vi "SysDef Launcher.vi"() -> ()   [LabVIEW 2014]
uses:
  NationalInstruments.VeriStand.Internal
  <vilib>/NI VeriStand/Execution/Workspace/NI_VS Workspace ExecutionAPI.lvlib
  <vilib>/NI Veristand/Execution/Project/NI_VS Project ExecutionAPI.lvlib
  NationalInstruments.VeriStand
panel:
  out "State":string
  in  "Stop":bool
  in  "Start":bool
  in  "System Definition File":path
  in  "Active Display":string(combo)
  in  "NIVS.App.Command":refnum<user-event>
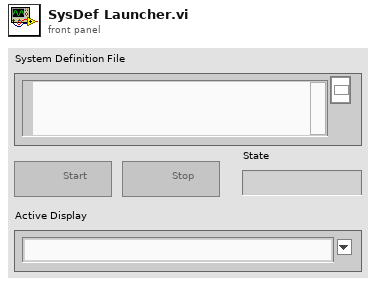
[diagram p1: front panel]
types:
  T1 = typedef "NI_VS Workspace ExecutionAPI.lvlib/WorkspaceAPI.ctl" = refnum<k24>
  T2 = typedef "NI_VS Workspace ExecutionAPI.lvlib/SystemStateEventRef.ctl" = cluster{"CustDatRef":refnum<user-event>, "EvtRef":refnum<k27>}
  T3 = typedef "NI_VS Workspace ExecutionAPI.lvlib/SystemStateRegEventRef.ctl" = refnum<event-registration>
  T4 = cluster{"Event Registration Refnum":refnum<event-registration>, "SystemChangeEventRef":T3}
  T5 = enum8{"Enabled", "Disabled", "Disabled and Grayed Out"}
  T6 = typedef "NI_VS Project ExecutionAPI.lvlib/Project Ref.ctl" = refnum<k24>
  T7 = typedef "NI_VS Workspace ExecutionAPI.lvlib/SystemState.ctl" = u8
  T8 = enum32{"invalid app kind", "Development System", "Run Time System", "Student Edition", "Embedded LabVIEW", "Evaluation", "Custom"}
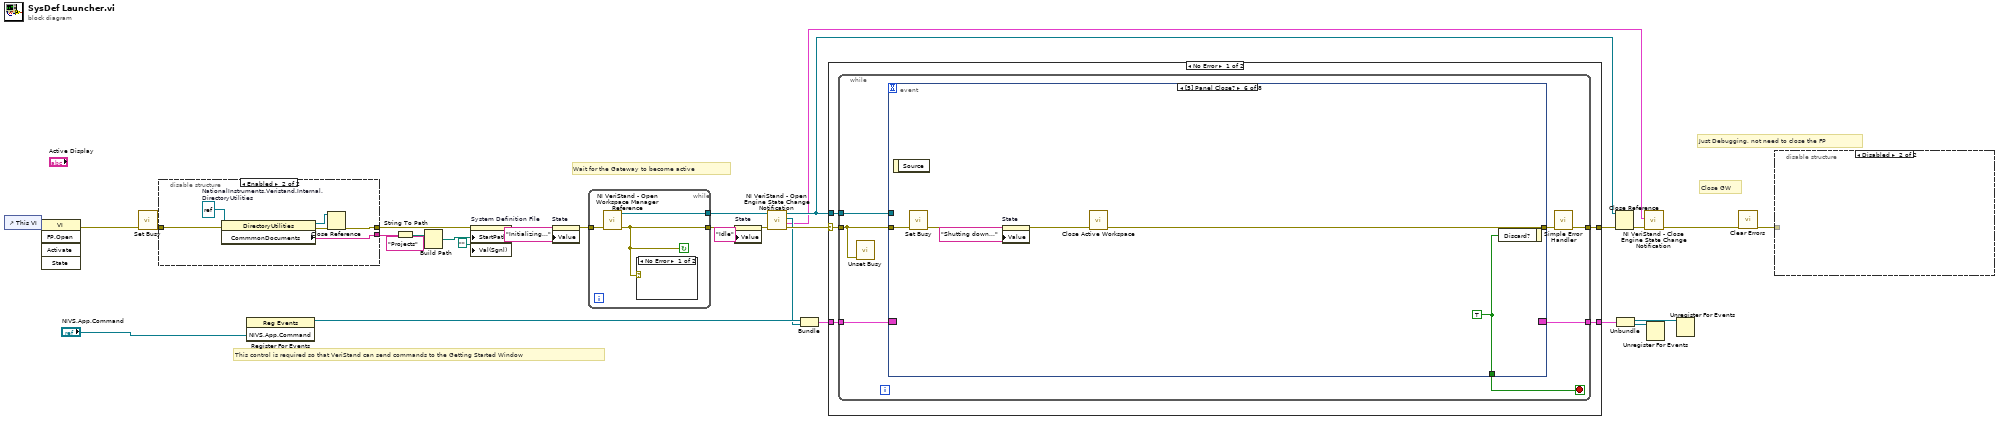
[diagram p0: block diagram]
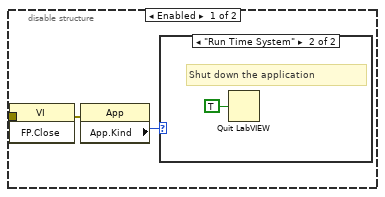
[diagram p2: hidden frame]
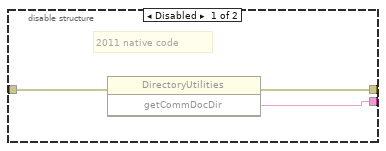
[diagram p4: hidden frame]
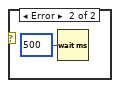
[diagram p5: hidden frame]
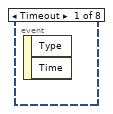
[diagram p6: hidden frame]
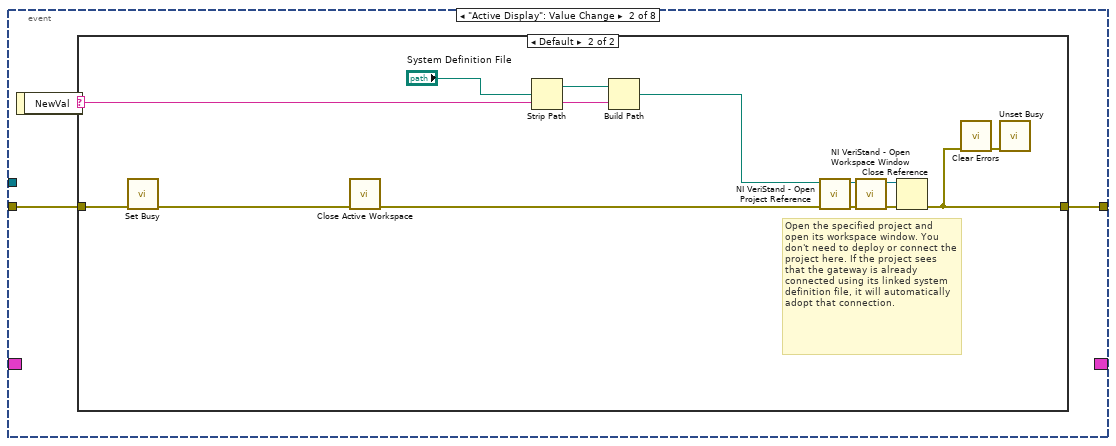
[diagram p7: hidden frame]
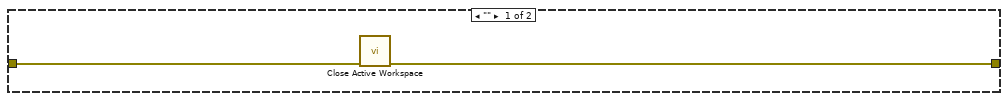
[diagram p8: hidden frame]
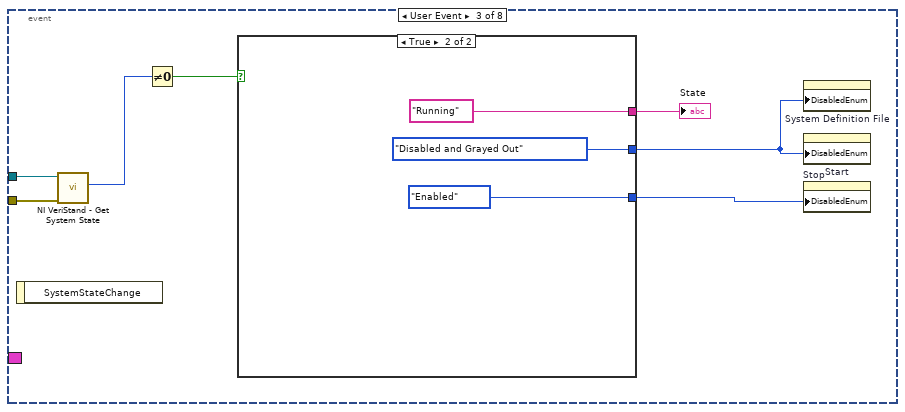
[diagram p9: hidden frame]
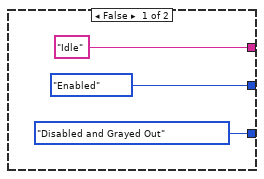
[diagram p10: hidden frame]
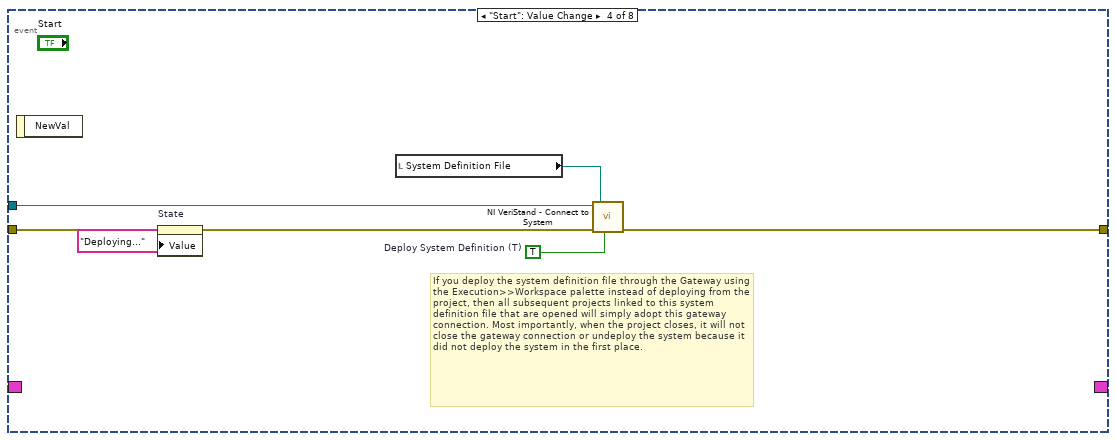
[diagram p11: hidden frame]
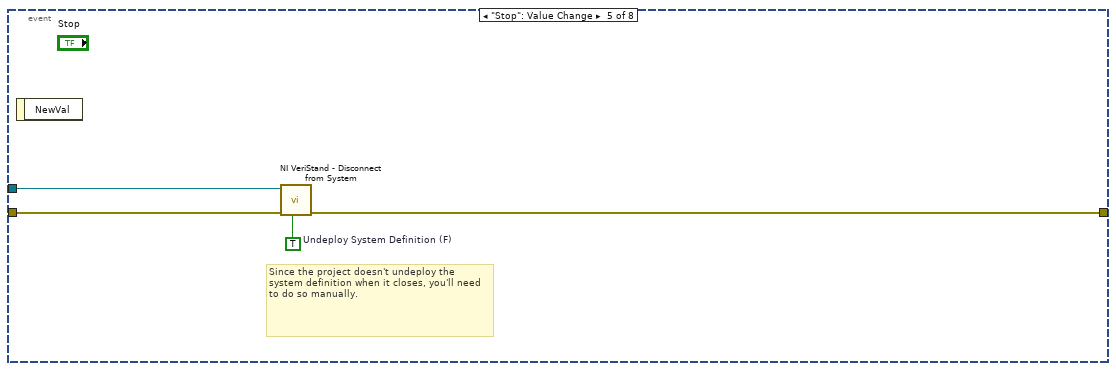
[diagram p12: hidden frame]
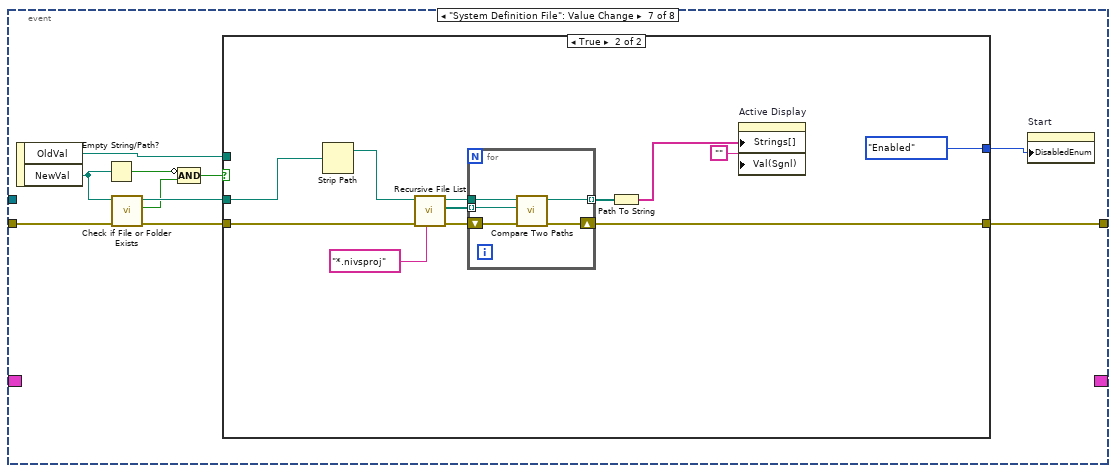
[diagram p13: hidden frame]
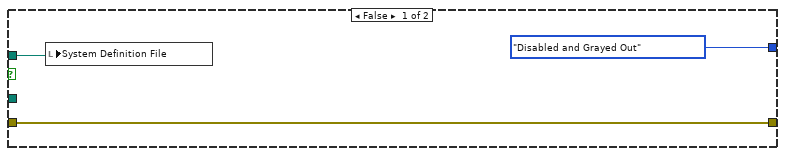
[diagram p14: hidden frame]
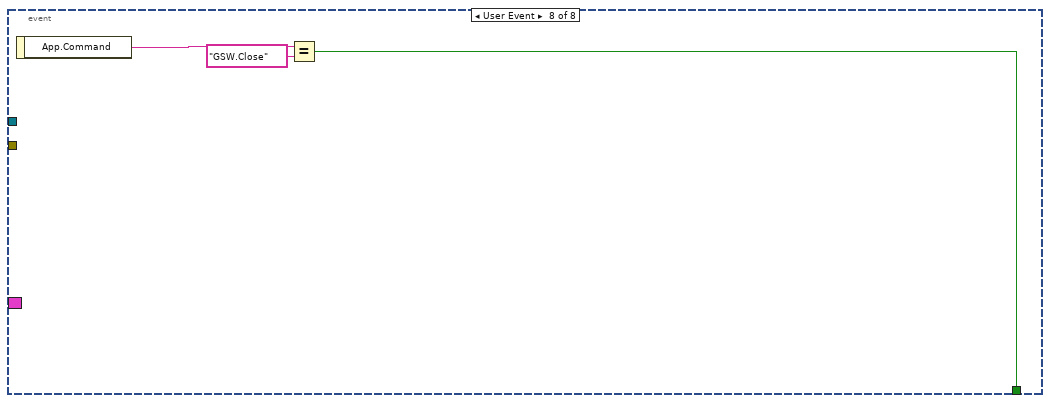
[diagram p15: hidden frame]
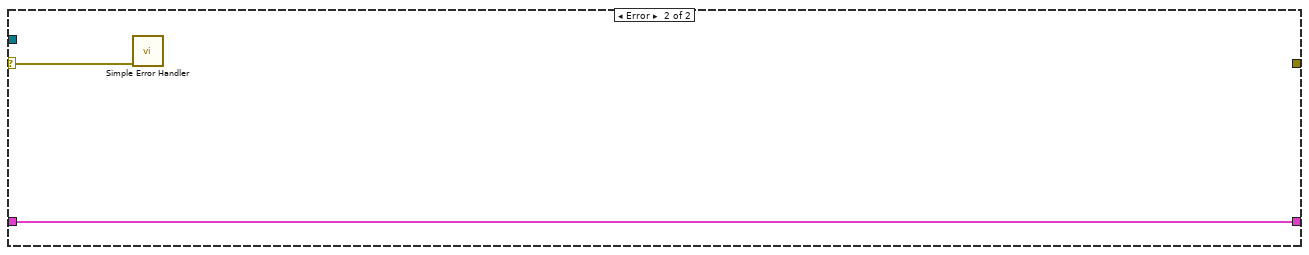
[diagram p16: hidden frame]
diagram:
  # "Close GW"
  # "Just Debugging, not need to close the FP"
  # "This control is required so that VeriStand can send commands to the Getting Started Window"
  # "Wait for the Gateway to become active"
  n1 = control-ref of="This VI"() -> (w29:refnum<vi>)
  n2 = invoke class="VI" method="FP.Open"(reference=w29) -> (error out=w2:errorcluster)  [unwired: 4 in, 4 out]
  n3 = call <vilib>:"Set Busy.vi"("error in (no error)"=w2) -> ("error out"=w4:errorcluster)  [unwired: 9 in, 1 out]
  n4 = disable-structure shown="Enabled" {
    disable-tunnel: [w33 w36] -> w27
    disable-tunnel: [w32 w38] -> w5
    disable-tunnel: w4 -> [w31 w35]
    frame Disabled {
      # "2011 native code"
      n5 = invoke class="DirectoryUtilities" method="getCommDocDir"(error in=w31) -> (error out=w32:errorcluster, "getCommDocDir"=w33:string)  [unwired: 2 in, 1 out]
    }
    frame Enabled {
      w34 = refnum<k24> refnum  # NationalInstruments.Veristand.Internal.DirectoryUtilities
      n6 = property class="DirectoryUtilities"(reference=w34, error in=w35) -> (reference out=w39:refnum<k24>, error out=w37:errorcluster, "CommmonDocuments"=w36:string)
      n7 = Close Reference(reference=w39, error in (no error)=w37) -> (error out=w38:errorcluster)
    }
  }
  n8 = register-events("NIVS.App.Command") -> (reference out=w21:refnum<event-registration>)  [unwired: 2 in, 1 out]
  n9 = String To Path(string=w27) -> (path=w26:path)
  n10 = Build Path(base path=w26, name or relative path="Projects") -> (appended path=w24:path)
  n11 = property on="System Definition File" class="Path"(error in=w5, "StartPath"=w24, "Val(Sgnl)"=path "") -> (error out=w11:errorcluster)  [unwired: 1 in, 1 out]
  n12 = property on="State" class="Str"(error in=w11, "Value"="Initializing..." ("State")) -> (error out=w10:errorcluster)  [unwired: 1 in, 1 out]
  n13 = while {
    tunnel: w10 -> [w42]
    tunnel: [w41] -> w22
    tunnel: [w40] -> w7
    stop <- w40 continue-if-true
    n14 = call <vilib>:"NI VeriStand - Open Workspace Manager Reference.vi"("error in (no error)"=w42) -> ("error out"=w40:errorcluster, "WorkspaceManager"=w41:T1)  [unwired: 9 in]
    n15 = case shown="No Error" w40 {
      frame No Error {
      }
      frame Error {
        n16 = Wait (ms)(milliseconds to wait=u32 500) -> ()  [unwired: 1 out]
      }
    }
  }
  n17 = property on="State" class="Str"(error in=w7, "Value"="Idle" ("State")) -> (error out=w6:errorcluster)  [unwired: 1 in, 1 out]
  n18 = call <vilib>:"NI VeriStand - Open Engine State Change Notification.vi"("error in (no error)"=w6, "WorkspaceManager in"=w22) -> ("error out"=w30:errorcluster, "SystemStateRefs"=w14:T2, "SystemChangeEventRef"=w19:T3, "WorkspaceManager out"=w18:T1)  [unwired: 6 in]
  n19 = Bundle("Event Registration Refnum"=w21, "SystemChangeEventRef"=w19) -> (w20:T4)  [unwired: 1 in]
  n20 = case shown="No Error" w30 {
    selector: w30 -> [w47 w137]
    tunnel: [w48 _] -> w23
    tunnel: w20 -> [w46 w138]
    tunnel: [w45 w138] -> w17
    tunnel: w18 -> [w44 _]
    frame No Error {
      n21 = while {
        tunnel: [w53] -> w48
        tunnel: w47 -> [w49]
        tunnel: w46 -> [w52]
        tunnel: [w51] -> w45
        tunnel: w44 -> [w50]
        stop <- w55 stop-if-true
        n22 = call <vilib>:"Unset Busy.vi"("error in (no error)"=w49) -> ()  [unwired: 10 in, 1 out]
        n23 = event shown="[5] Panel Close?" {
          selector: w52 -> [_ _ _ _ _ _ _ _]
          dyn-events: [_ _ _ _ _ _ _ _] -> w51
          timeout: _ -> [_ _ _ _ _ _ _ _]
          tunnel: [_ _ _ _ _ w103 _ w134] -> w55
          tunnel: [_ w58 _ w90 w94 w98 w105 _] -> w54
          tunnel: w49 -> [_ w57 w79 w88 w96 w100 w113 _]
          tunnel: w50 -> [_ _ w80 w91 w95 _ _ _]
          event Timeout {
            n24 = event-data() -> ()  [unwired: 1 in, 2 out]
          }
          event "Active Display": Value Change {
            n25 = event-data() -> ("NewVal"=w56:string)  [unwired: 1 in]
            n26 = case shown="Default" w56 {
              selector: w56 -> [_ w66]
              tunnel: [w59 w63] -> w58
              tunnel: w57 -> [w60 w65]
              frame "" {
                n27 = call "Close Active Workspace.vi"("error in (no error)"=w60) -> ("error out"=w59:errorcluster)  [unwired: 10 in]
              }
              frame Default {
                # "Open the specified project and open its workspace window. You don't need to deploy or connect the project here. If the project sees that the gateway is already connected using its linked system definition file, it will automatically adopt that connection."
                n28 = call <vilib>:"Set Busy.vi"("error in (no error)"=w65) -> ("error out"=w62:errorcluster)  [unwired: 9 in, 1 out]
                n29 = call "Close Active Workspace.vi"("error in (no error)"=w62) -> ("error out"=w61:errorcluster)  [unwired: 10 in]
                n30 = Strip Path(path="System Definition File") -> (stripped path=w70:path)  [unwired: 1 out]
                n31 = Build Path(base path=w70, name or relative path=w66) -> (appended path=w69:path)
                n32 = call <vilib>:"NI VeriStand - Open Project Reference.vi"("error in (no error)"=w61, "Project File Path"=w69) -> ("error out"=w68:errorcluster, "Project Ref"=w67:T6)  [unwired: 8 in]
                n33 = call <vilib>:"NI VeriStand - Open Workspace Window.vi"("error in (no error)"=w68, "Project Ref in"=w67) -> ("error out"=w73:errorcluster, "Project Ref out"=w72:T6)  [unwired: 8 in]
                n34 = Close Reference(reference=w72, error in (no error)=w73) -> (error out=w63:errorcluster)
                n35 = call <vilib>:"Clear Errors.vi"("error in (no error)"=w63) -> ("error out"=w64:errorcluster)  [unwired: 5 in, 1 out]
                n36 = call <vilib>:"Unset Busy.vi"("error in (no error)"=w64) -> ()  [unwired: 10 in, 1 out]
              }
            }
          }
          event User Event {
            n37 = event-data() -> ()  [unwired: 1 in, 1 out]
            n38 = call <vilib>:"NI VeriStand - Get System State.vi"("error in (no error)"=w79, "WorkspaceManager in"=w80) -> ("System State"=w78:T7)  [unwired: 5 in, 4 out]
            n39 = Not Equal To 0?(x=w78) -> (x != 0?=w77:bool)
            n40 = case shown="True" w77 {
              tunnel: ["Idle" ("State") "Running" ("State")] -> w74
              tunnel: [T5."Enabled" ("Disabled") T5."Disabled and Grayed Out" ("Disabled")] -> w75
              tunnel: [T5."Disabled and Grayed Out" ("Disabled") T5."Enabled" ("Disabled")] -> w76
              frame False {
              }
              frame True {
              }
            }
            "State" <- w74
            n41 = property on="System Definition File" class="Path"("DisabledEnum"=w75) -> ()  [unwired: 2 in, 2 out]
            n42 = property on="Start" class="Bool"("DisabledEnum"=w75) -> ()  [unwired: 2 in, 2 out]
            n43 = property on="Stop" class="Bool"("DisabledEnum"=w76) -> ()  [unwired: 2 in, 2 out]
          }
          event "Start": Value Change {
            w93 = TRUE  # Deploy System Definition (T)
            # "If you deploy the system definition file through the Gateway using the Execution>>Workspace palette instead of deploying from the project, then all subsequent projects linked to this system definition file that are opened will simply adopt this gateway connection. Most importantly, when the project closes, it will not close the gateway connection or undeploy the system because it did not deploy the system in the first place."
            n44 = event-data() -> ()  [unwired: 1 in, 1 out]
            n45 = property on="State" class="Str"(error in=w88, "Value"="Deploying..." ("State")) -> (error out=w87:errorcluster)  [unwired: 1 in, 1 out]
            n46 = local read "System Definition File"() -> (w92:path)
            n47 = call <vilib>:"NI VeriStand - Connect to System.vi"("Deploy System Definition (T)"=w93, "error in (no error)"=w87, "System Definition File (.nivssdf)"=w92, "WorkspaceManager in"=w91) -> ("error out"=w90:errorcluster)  [unwired: 6 in, 1 out]
          }
          event "Stop": Value Change {
            w97 = TRUE  # Undeploy System Definition (F)
            # "Since the project doesn't undeploy the system definition when it closes, you'll need to do so manually."
            n48 = event-data() -> ()  [unwired: 1 in, 1 out]
            n49 = call <vilib>:"NI VeriStand - Disconnect from System.vi"("Undeploy System Definition (F)"=w97, "error in (no error)"=w96, "WorkspaceManager in"=w95) -> ("error out"=w94:errorcluster)  [unwired: 7 in, 1 out]
          }
          event Panel Close? {
            w103 = TRUE
            n50 = event-data() -> ()  [unwired: 1 in, 1 out]
            n51 = call <vilib>:"Set Busy.vi"("error in (no error)"=w100) -> ("error out"=w99:errorcluster)  [unwired: 9 in, 1 out]
            n52 = property on="State" class="Str"(error in=w99, "Value"="Shutting down..." ("State")) -> (error out=w101:errorcluster)  [unwired: 1 in, 1 out]
            n53 = call "Close Active Workspace.vi"("error in (no error)"=w101) -> ("error out"=w98:errorcluster)  [unwired: 10 in]
            n54 = event-data("Discard?"=w103) -> ()  [unwired: 1 in, 1 out]
          }
          event "System Definition File": Value Change {
            n55 = event-data() -> ("OldVal"=w106:path, "NewVal"=w110:path)  [unwired: 1 in]
            n56 = Empty String/Path?(string/path=w110) -> (empty?=w108:bool)
            n57 = call <vilib>:"Check if File or Folder Exists.vi"("error in (no error)"=w113, "path"=w110) -> ("error out"=w112:errorcluster, "file or folder exists?"=w109:bool, "dup path"=w111:path)  [unwired: 7 in]
            n58 = Compound Arithmetic op=AND(invert w108, w109) -> (w107:bool)
            n59 = case shown="True" w107 {
              tunnel: w112 -> [w115 w128]
              tunnel: w111 -> [_ w127]
              tunnel: w106 -> [w116 _]
              tunnel: [w115 w118] -> w105
              tunnel: [T5."Disabled and Grayed Out" ("Disabled") T5."Enabled" ("Disabled")] -> w104
              frame False {
                n60 = local write "System Definition File"(w116) -> ()
              }
              frame True {
                n61 = Strip Path(path=w127) -> (stripped path=w126:path)  [unwired: 1 out]
                n62 = call <vilib>:"Recursive File List.vi"("pattern"="*.nivsproj", "error in (no error)"=w128, "Folder Path"=w126) -> ("error out"=w124:errorcluster, "All Files in Dir"=w123:path[], "dup Folder Path"=w122:path)  [unwired: 4 in, 2 out]
                n63 = for {
                  tunnel: w123 -> [w132] mode=indexing
                  tunnel: w122 -> [w131]
                  tunnel: [w130] -> w121 mode=indexing
                  shift-right: [w129] -> w118
                  shift-left: w124 -> [w133]
                  n64 = call <vilib>:"Compare Two Paths.vi"("error in (no error)"=w133, "Path 2"=w132, "Path 1"=w131) -> ("error out"=w129:errorcluster, "Relative Path from 1 to 2"=w130:path)  [unwired: 5 in, 2 out]
                }
                n65 = Path To String(path=w121) -> (string=w120:string[])
                n66 = property on="Active Display" class="CmbBox"("Strings[]"=w120, "Val(Sgnl)"="") -> ()  [unwired: 2 in, 2 out]
              }
            }
            n67 = property on="Start" class="Bool"("DisabledEnum"=w104) -> ()  [unwired: 2 in, 2 out]
          }
          event User Event {
            n68 = event-data() -> ("App.Command"=w136:string)  [unwired: 1 in]
            n69 = Equal?(x=w136, y="GSW.Close") -> (x = y?=w134:bool)
          }
        }
        n70 = call <vilib>:"Simple Error Handler.vi"("error in (no error)"=w54) -> ("error out"=w53:errorcluster)  [unwired: 4 in, 4 out]
      }
    }
    frame Error {
      n71 = call <vilib>:"Simple Error Handler.vi"("error in (no error)"=w137) -> ()  [unwired: 4 in, 5 out]
    }
  }
  n72 = Close Reference(reference=w18, error in (no error)=w23) -> (error out=w12:errorcluster)
  n73 = Unbundle(w17) -> ("Event Registration Refnum"=w15:refnum<event-registration>, "SystemChangeEventRef"=w16:T3)
  n74 = call <vilib>:"NI VeriStand - Close Engine State Change Notification.vi"("error in (no error)"=w12, "SystemStateRefs"=w14) -> ("error out"=w1:errorcluster)  [unwired: 9 in]
  n75 = Unregister For Events(event registration refnum=w16) -> ()  [unwired: 1 in, 1 out]
  n76 = Unregister For Events(event registration refnum=w15) -> ()  [unwired: 1 in, 1 out]
  n77 = call <vilib>:"Clear Errors.vi"("error in (no error)"=w1) -> ("error out"=w3:errorcluster)  [unwired: 5 in, 1 out]
  n78 = disable-structure shown="Disabled" {
    disable-tunnel: w3 -> [w141 _]
    frame Enabled {
      n79 = invoke class="VI" method="FP.Close"(error in=w141) -> (error out=w140:errorcluster)  [unwired: 2 in, 2 out]
      n80 = property class="App"(error in=w140) -> ("App.Kind"=w139:T8)  [unwired: 1 in, 2 out]
      n81 = case shown="\"Run Time System\"" w139 {
        frame Default {
        }
        frame "Run Time System" {
          # "Shut down the application"
          n82 = Quit LabVIEW(quit? (T)=TRUE) -> ()
        }
      }
    }
    frame Disabled {
    }
  }
